vi "Get Data I16_32.vi"(8 "error in (no error)":errorcluster, 11 "RFSoC Driver in":refnum<class "RFSoC Driver.lvclass">) -> (0 "error out":errorcluster, 1 "I32 data out":i32[][](array[numeric]), 2 "I16 data out":i16[][](array[numeric]), 3 "RFSoC Driver out":refnum<class "RFSoC Driver.lvclass">, 4 "Finished":bool, 5 "Current read position":i32)   [LabVIEW 2019, in "RFSoC Driver.lvclass"]
uses:
  RFSoC Driver.lvclass
  C:/GitHub/NHMFL_Core/Libraries/Instruments/Pulse Driver/Pulse Driver.lvclass
  Pulse Driver/Pulse Driver.lvclass/Pulse Driver.ctl
  RFSoC Driver.lvclass/RFSoC Driver.ctl
  Pulse Driver/Read Samples per read.vi
  Read Mixer.vi
panel:
  out "Record responce":string[](array[string])
  out "Extra data out":string
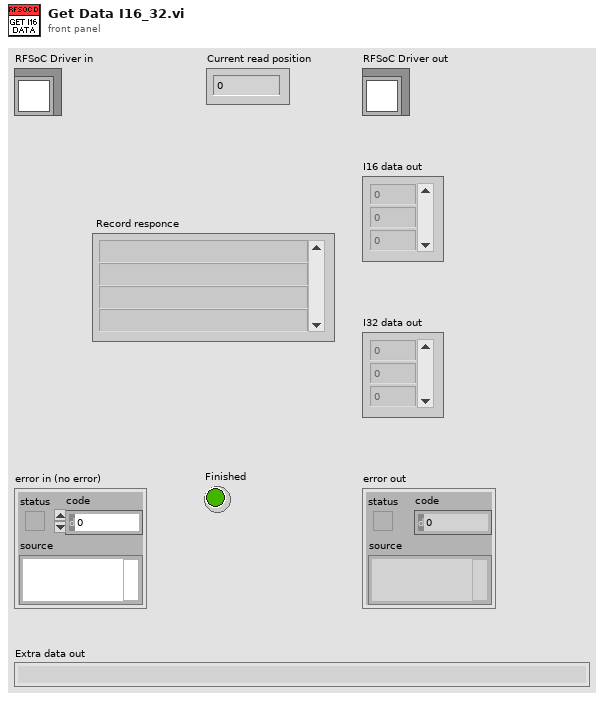
[diagram p1: front panel]
types:
  T1 = enum16{"big-endian, network order", "native, host order", "little-endian"}
  T2 = enum16{"Standard", "Buffered", "CRLF", "Immediate"}
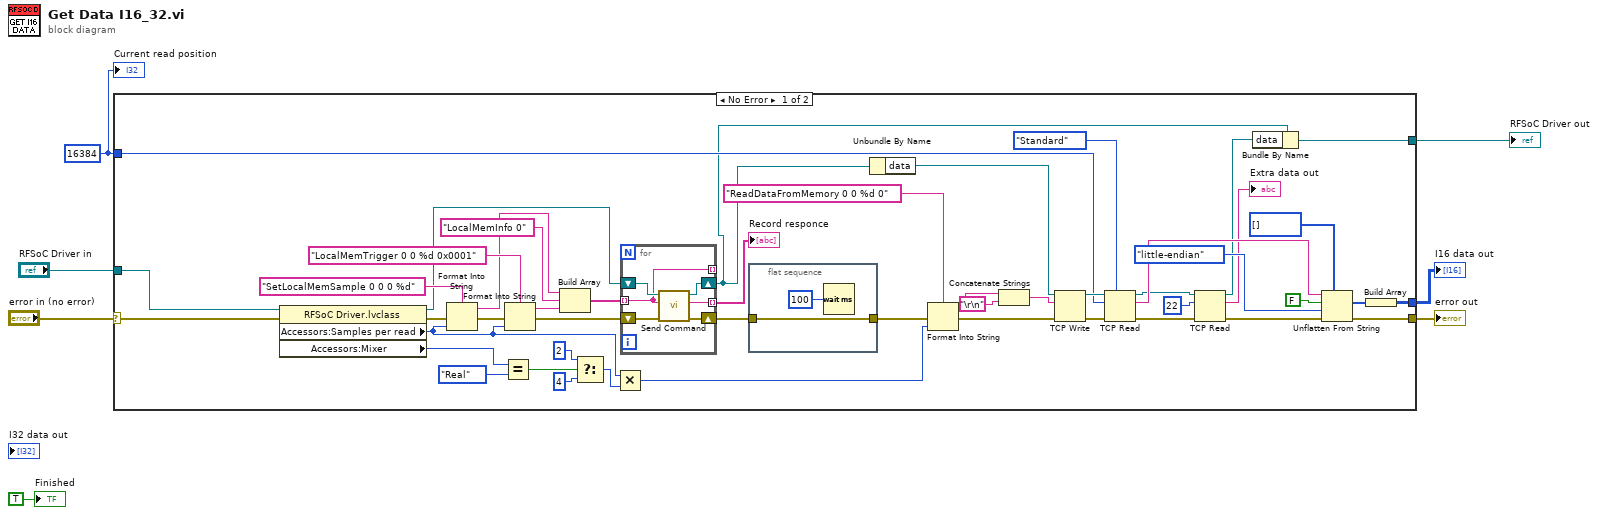
[diagram p0: block diagram]
diagram:
  w2 = 16384
  n1 = case shown="No Error" "error in (no error)" {
    selector: "error in (no error)" -> [w52 w65]
    tunnel: [w42 w65] -> w4
    tunnel: [w49 w64] -> w1
    tunnel: "RFSoC Driver in" -> [w33 w64]
    tunnel: w2 -> [w47 _]
    tunnel: [w40 _] -> w5
    frame No Error {
      n2 = property class="RFSoC Driver.lvclass"(reference=w33, error in=w52) -> (reference out=w22:refnum<class "RFSoC Driver.lvclass">, error out=w31:errorcluster, "Accessors:Samples per read"=w12:i32, "Accessors:Mixer"=w14:enum16{"Real", "I/Q"})
      n3 = Format Into String(format string="SetLocalMemSample 0 0 0 %d", error in=w31, w12) -> (resulting string=w28:string, error out=w30:errorcluster)  [unwired: 1 in]
      n4 = Equal?(x=w14, y=enum16{"Real", "I/Q"}."Real" ("Mixer")) -> (x = y?=w18:bool)
      n5 = Format Into String(format string="LocalMemTrigger 0 0 %d 0x0001", error in=w30, w12) -> (resulting string=w27:string, error out=w25:errorcluster)  [unwired: 1 in]
      n6 = Build Array(w28, "LocalMemInfo 0", w27) -> (w23:string[])
      n7 = Select(t=2 ("Binary sample width"), s=w18, f=4 ("Binary sample width")) -> (s? t:f=w13:i32)
      n8 = Multiply(x=w12, y=w13) -> (x*y=w11:i32)
      n9 = for {
        shift-right: [w61] -> w21
        shift-left: w22 -> [w63]
        shift-right: [w60] -> w24
        shift-left: w25 -> [w62]
        tunnel: [w58] -> _ mode=indexing
        tunnel: [w59] -> w20 mode=indexing
        tunnel: w23 -> [w58] mode=indexing
        n10 = call-dynamic "Send Command.vi"("error in (no error)"=w62, "Command"=w58, "RFSoC Driver in"=w63) -> ("error out"=w60:errorcluster, "Responce"=w59:string, "RFSoC Driver out"=w61:refnum<class "RFSoC Driver.lvclass">)  [unwired: 6 in]
      }
      "Record responce" <- w20
      n11 = flat-sequence {
        tunnel: w24 -> [w57]
        tunnel: [w57] -> w9
        frame #0 {
          n12 = Wait (ms)(milliseconds to wait=u32 100) -> ()  [unwired: 1 out]
        }
      }
      n13 = Unbundle By Name(w21) -> ("data"=w55:refnum<k5>)
      n14 = Format Into String(format string="ReadDataFromMemory 0 0 %d 0", error in=w9, w11) -> (resulting string=w10:string, error out=w8:errorcluster)  [unwired: 1 in]
      n15 = Concatenate Strings(w10, "\r\n") -> (w53:string)
      n16 = TCP Write(connection ID=w55, data in=w53, error in (no error)=w8) -> (connection ID out=w50:refnum<k5>, error out=w51:errorcluster)  [unwired: 1 in, 1 out]
      n17 = TCP Read(connection ID=w50, bytes to read=w47, error in (no error)=w51, 7:T2."Standard" ("mode (standard)")) -> (connection ID out=w37:refnum<k5>, data out=w46:string, error out=w39:errorcluster)  [unwired: 1 in]
      n18 = TCP Read(connection ID=w37, bytes to read=22, error in (no error)=w39) -> (connection ID out=w36:refnum<k5>, data out=→"Extra data out":string, error out=w38:errorcluster)  [unwired: 2 in]
      n19 = Bundle By Name(cluster=w21, "data"=w36) -> (w49:refnum<class "RFSoC Driver.lvclass">)
      n20 = Unflatten From String(type=i16[] [], binary string=w46, data includes array or string size? (T)=FALSE, byte order (0:big-endian, network order)=T1."little-endian", error in (no error)=w38) -> (value=w41:i16[], error out=w42:errorcluster)  [unwired: 1 out]
      n21 = Build Array(w41) -> (w40:i16[][])
    }
    frame Error {
    }
  }
  "error out" <- w4
  "RFSoC Driver out" <- w1
  "I16 data out" <- w5
  "Current read position" <- w2
  "Finished" <- TRUE ("Finished")
